vi "2400_2182a_4probe.vi"() -> ()   [LabVIEW 2021]
uses:
  <instrlib>/Keithley 24XX/Public/Data/Read (Single Point).vi
  <instrlib>/Keithley 2182/Keithley 2182.lvlib
  <instrlib>/Keithley 24XX/Keithley 24XX.lvlib
panel:
  in  "Settling Delay":dbl=2.0
  out "New file path 2":path
  in  "Folder to save file to 2":path
  out "XY Graph":cluster{sgl[], "Measurements":dbl[]}(graph)
  in  "Timeout (10000 ms)":i32=10000 format="%#.6g"
  in  "VISA 2400 Sourcemeter":refnum<visa-resource-name>
  in  "VISA NanoVoltmeter":refnum<visa-resource-name>
  in  "Integration Rate (5)":dbl=5.0
  in  "Range Value (12)":dbl=12.0
  in  "Voltage Resolution (8)":i32=8
  in  "Measurement (0: Voltage Channel 1)":i32(ring) items=["Voltage Channel 1", "Voltage Channel 2", "Temperature Channel 1", "Temperature Channel 2"]
  in  "Number of Points (5)":u32=5
  in  "Source Mode  (0: Voltage)":u16(ring) items=["Voltage", "Current"]
  in  "Maximum Amplitude (2)":dbl=2.0
  in  "Minimum Amplitude (1)":dbl=1.0
  in  "Compliance  Level (0.1)":dbl=0.1
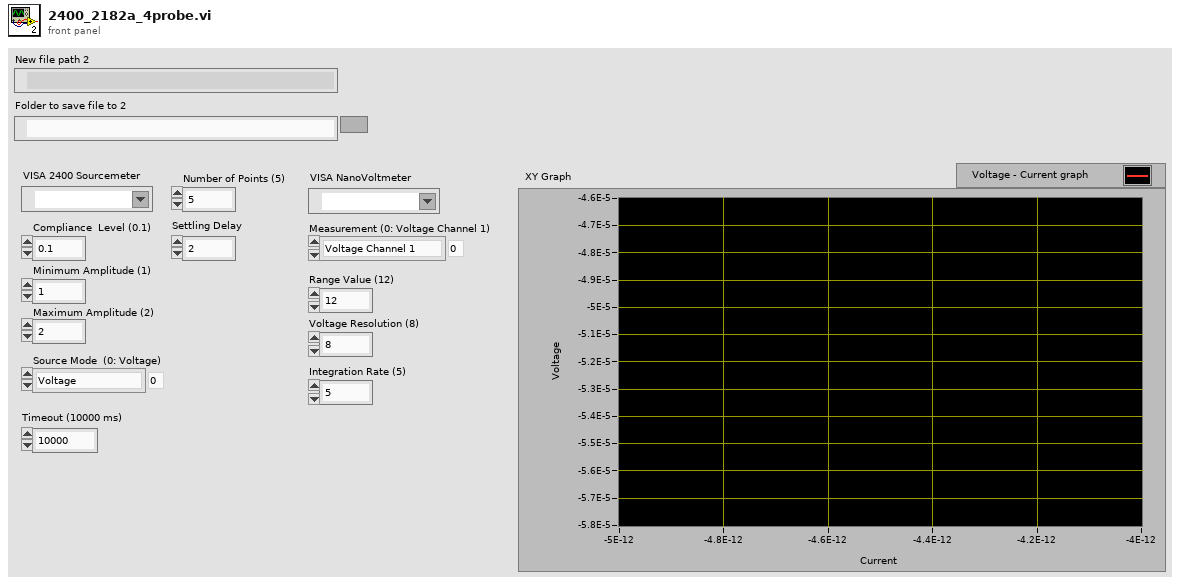
[diagram p1: front panel]
types:
  T1 = enum16{"open", "replace", "create", "open or create", "replace or create", "replace or create with confirmation"}
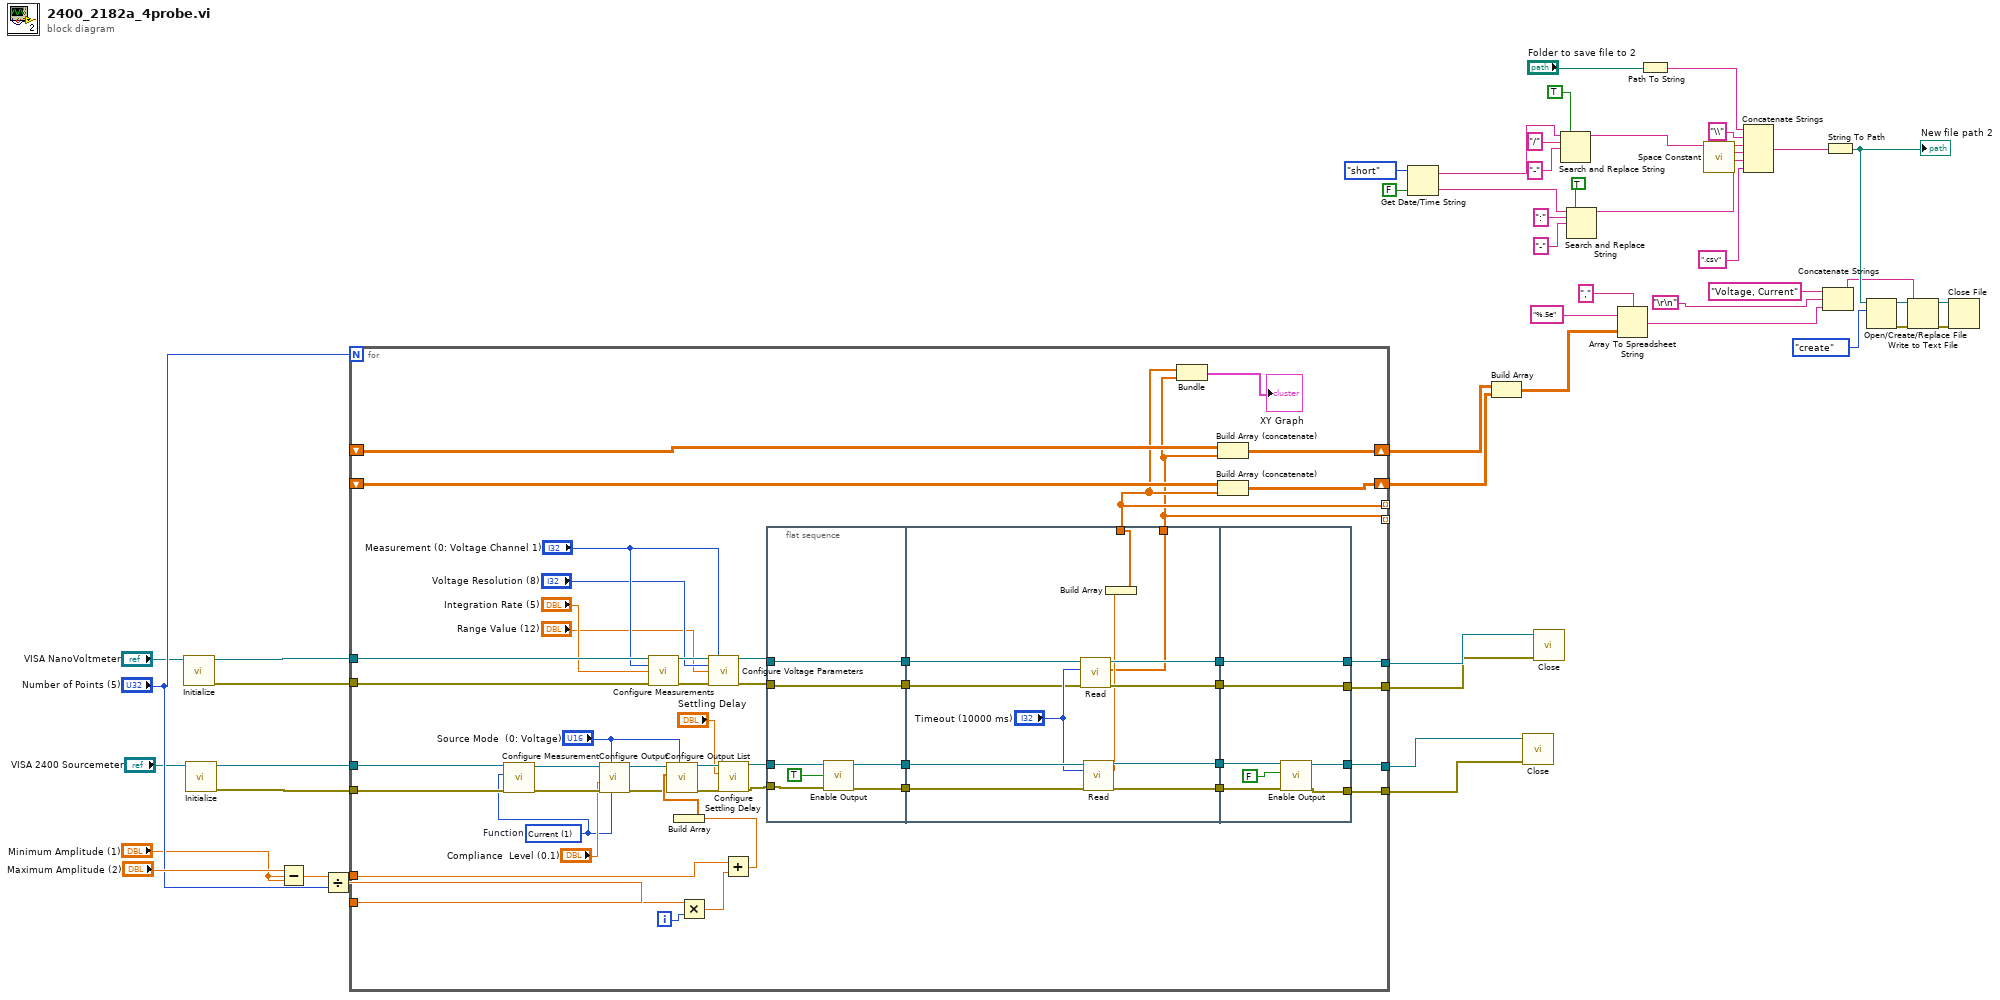
[diagram p0: block diagram]
diagram:
  n1 = call <instrlib>:"Initialize.vi"("VISA resource name"="VISA NanoVoltmeter") -> ("error out"=w1:errorcluster, "VISA resource name out"=w2:refnum<visa-resource-name>)  [unwired: 9 in]
  n2 = call <instrlib>:"Initialize.vi"("VISA resource name"="VISA 2400 Sourcemeter") -> ("error out"=w3:errorcluster, "VISA resource name out"=w4:refnum<visa-resource-name>)  [unwired: 9 in]
  n3 = Subtract(x="Maximum Amplitude (2)", y="Minimum Amplitude (1)") -> (x-y=w47:dbl)
  n4 = Divide(x=w47, y="Number of Points (5)") -> (x/y=w45:dbl)
  n5 = for {
    N: "Number of Points (5)" -> [_]
    tunnel: w45 -> [w79]
    tunnel: [w87] -> w42
    tunnel: [w89] -> w41
    tunnel: [w92] -> w40
    tunnel: [w91] -> w39
    shift-right: [w83] -> w37
    shift-left: _ -> [w84]
    shift-right: [w81] -> w36
    shift-left: _ -> [w82]
    tunnel: [w75] -> _ mode=indexing
    tunnel: [w74] -> _ mode=indexing
    tunnel: "Minimum Amplitude (1)" -> [w80]
    tunnel: w4 -> [w64]
    tunnel: w3 -> [w63]
    tunnel: w2 -> [w61]
    tunnel: w1 -> [w60]
    i -> [w78]
    w55 = u16 1 items=["Volts", "Current", "Resistance"]  # Function
    n6 = call <instrlib>:"Configure Measurement.vi"("error in (no error)"=w63, "Function (0: Volts)"=w55, "VISA resource name"=w64) -> ("error out"=w67:errorcluster, "VISA resource name out"=w68:refnum<visa-resource-name>)  [unwired: 7 in]
    n7 = call <instrlib>:"Configure Output.vi"("Output Type  (0: Immediate)"=w55, "Source Mode  (0: Voltage)"="Source Mode  (0: Voltage)", "error in (no error)"=w67, "Compliance  Level (0.1)"="Compliance  Level (0.1)", "VISA resource name"=w68) -> ("error out"=w65:errorcluster, "VISA resource name out"=w66:refnum<visa-resource-name>)  [unwired: 5 in]
    n8 = call <instrlib>:"Configure Measurements.vi"("VISA resource name"=w61, "Measurement (0: Voltage Channel 1)"="Measurement (0: Voltage Channel 1)", "Integration Rate (5)"="Integration Rate (5)", "error in (no error)"=w60) -> ("VISA resource name out"=w72:refnum<visa-resource-name>, "error out"=w71:errorcluster)  [unwired: 10 in]
    n9 = Multiply(x=w79, y=w78) -> (x*y=w77:dbl)
    n10 = call <instrlib>:"Configure Voltage Parameters.vi"("VISA resource name"=w72, "Measurement (1: Voltage Channel 1)"="Measurement (0: Voltage Channel 1)", "Voltage Resolution (8)"="Voltage Resolution (8)", "Range Value (12)"="Range Value (12)", "error in (no error)"=w71) -> ("VISA resource name out"=w70:refnum<visa-resource-name>, "error out"=w69:errorcluster)  [unwired: 9 in]
    n11 = Add(x=w80, y=w77) -> (x+y=w76:dbl)
    n12 = Build Array(w76) -> (w93:dbl[])
    n13 = call <instrlib>:"Configure Output List.vi"("Source Mode  (0: Voltage)"="Source Mode  (0: Voltage)", "error in (no error)"=w65, "Output List"=w93, "VISA resource name"=w66) -> ("error out"=w51:errorcluster, "VISA resource name out"=w52:refnum<visa-resource-name>)  [unwired: 6 in]
    n14 = call <instrlib>:"Configure Settling Delay.vi"("error in (no error)"=w51, "Manual Settling Delay (0 sec)"="Settling Delay", "VISA resource name"=w52) -> ("error out"=w50:errorcluster, "VISA resource name out"=w53:refnum<visa-resource-name>)  [unwired: 7 in]
    n15 = flat-sequence {
      tunnel: [w104] -> w97
      tunnel: [w103] -> w95
      tunnel: w53 -> [w102]
      tunnel: w69 -> [w100]
      tunnel: [w100] -> w86
      tunnel: w70 -> [w99]
      tunnel: [w99] -> w85
      tunnel: w50 -> [w98]
      tunnel: w97 -> [w116]
      tunnel: [w115] -> w96
      tunnel: w95 -> [w114]
      tunnel: [w113] -> w94
      tunnel: [w111] -> w90
      tunnel: [w110] -> w88
      tunnel: w86 -> [w109]
      tunnel: w85 -> [w108]
      tunnel: [w105] -> w75
      tunnel: [w106] -> w74
      tunnel: w96 -> [w123]
      tunnel: w94 -> [w122]
      tunnel: [w120] -> w92
      tunnel: [w119] -> w91
      tunnel: [w118] -> w89
      tunnel: w90 -> [w118]
      tunnel: [w117] -> w87
      tunnel: w88 -> [w117]
      frame #0 {
        n16 = call <instrlib>:"Enable Output.vi"("error in (no error)"=w98, "Enable Output (T: Enable)"=TRUE, "VISA resource name"=w102) -> ("error out"=w103:errorcluster, "VISA resource name out"=w104:refnum<visa-resource-name>)  [unwired: 7 in]
      }
      frame #1 {
        n17 = call <instrlib>:"Read.vi"("error in (no error)"=w109, "Timeout(10000 ms)"="Timeout (10000 ms)", "VISA resource name"=w108) -> ("error out"=w111:errorcluster, "Measurements"=w106:dbl[], "VISA resource name out"=w110:refnum<visa-resource-name>)  [unwired: 5 in, 1 out]
        n18 = call-poly <instrlib>:"Read.vi"("VISA resource name"=w116, "Timeout (10000 ms)"="Timeout (10000 ms)", "error in (no error)"=w114) -> ("VISA resource name out"=w115:refnum<visa-resource-name>, "Current"=w107:sgl, "error out"=w113:errorcluster)  [unwired: 6 in, 4 out]
        n19 = Build Array(w107) -> (w105:sgl[])
      }
      frame #2 {
        n20 = call <instrlib>:"Enable Output.vi"("error in (no error)"=w122, "Enable Output (T: Enable)"=FALSE, "VISA resource name"=w123) -> ("error out"=w119:errorcluster, "VISA resource name out"=w120:refnum<visa-resource-name>)  [unwired: 7 in]
      }
    }
    n21 = Bundle(w75, "Measurements"=w74) -> (→"XY Graph":cluster{sgl[], "Measurements":dbl[]})  [unwired: 1 in]
    n22 = Build Array (concatenate)(w84, w74) -> (w83:dbl[][])
    n23 = Build Array (concatenate)(w82, w75) -> (w81:sgl[][])
  }
  n24 = Get Date/Time String(date format (0)=enum16{"short", "long", "abbreviated"}."short", want seconds? (F)=FALSE) -> (date string=w7:string, time string=w19:string)  [unwired: 1 in]
  n25 = Build Array(w37, w36) -> (w10:dbl[][][])
  n26 = call <instrlib>:"Close.vi"("error in (no error)"=w39, "VISA resource name"=w40) -> ()  [unwired: 9 in, 1 out]
  n27 = call <instrlib>:"Close.vi"("error in (no error)"=w41, "VISA resource name"=w42) -> ()  [unwired: 9 in, 1 out]
  n28 = Search and Replace String(replace all?=TRUE, input string=w7, search string="/" ("replace string (\"\")"), replace string="-" ("replace string (\"\")")) -> (result string=w6:string)  [unwired: 4 in, 3 out]
  n29 = Search and Replace String(replace all?=TRUE ("replace all? (F)"), input string=w19, search string=":" ("replace string (\"\")"), replace string="-" ("replace string (\"\")")) -> (result string=w23:string)  [unwired: 4 in, 3 out]
  n30 = Array To Spreadsheet String(delimiter (Tab)=",", array=w10, 3:"%.5e") -> (spreadsheet string=w12:string)
  n31 = Path To String(path="Folder to save file to 2") -> (string=w27:string)
  n32 = call <vilib>:"Space Constant.vi"() -> ("String"=w22:string)
  n33 = Concatenate Strings "Concatenate Strings"(w27, "\\" ("string"), w6, w22, w23, ".csv" ("string")) -> (w25:string)
  n34 = Concatenate Strings("Voltage, Current", "\r\n", w12) -> (w16:string)
  n35 = String To Path(string=w25) -> (path=w32:path)
  "New file path 2" <- w32
  n36 = Open/Create/Replace File(file path (use dialog)=w32, operation (0:open)=T1."create") -> (refnum out=w33:refnum<file>, error out=w34:errorcluster)  [unwired: 4 in, 1 out]
  n37 = Write to Text File(file (use dialog)=w33, text=w16, error in=w34) -> (refnum out=w30:refnum<file>, error out=w31:errorcluster)  [unwired: 1 in, 1 out]
  n38 = Close File(refnum=w30, error in=w31) -> ()  [unwired: 2 out]
